vi "MCListbox Controls.vi"(8 "error in":errorcluster, 9 "Item Names":string[][](array[string])=[["localhost", "DMM", "Closed"], ["localhost", "DC Power", "Closed"], ["localhost", "Digitizer", "Closed"]], 11 "MCListBox Ref":refnum<vi>) -> (0 "error out":errorcluster, 3 "dup MCListBox Ref":refnum<vi>)   [LabVIEW 2025, in "Config Tool.lvlib"]
uses:
  Config Tool.lvlib
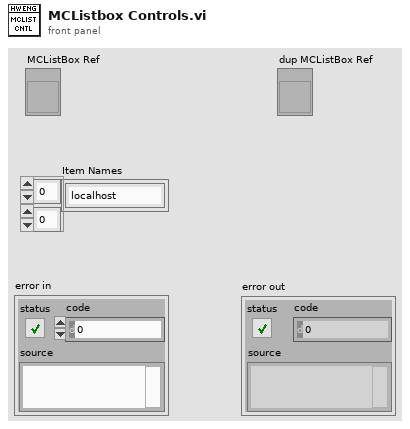
[diagram p1: front panel]
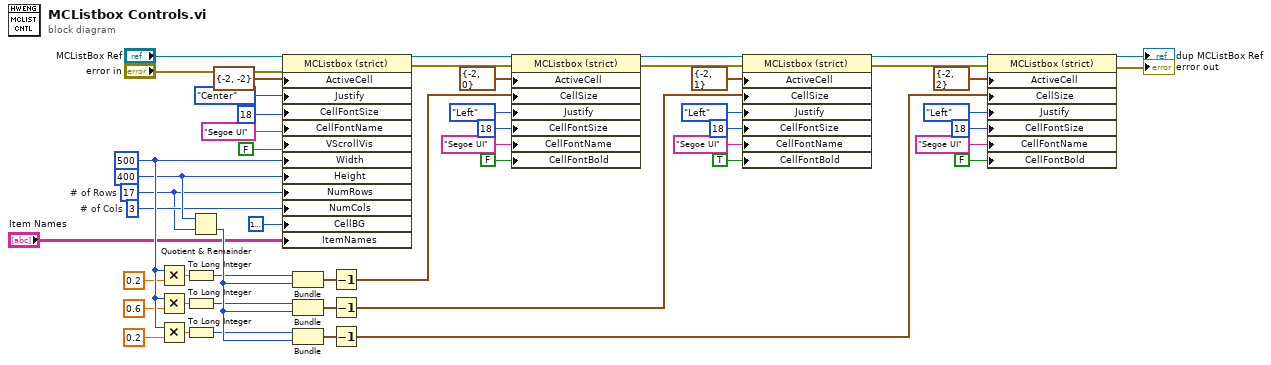
[diagram p0: block diagram]
diagram:
  w35 = u32 400
  w51 = u32 500
  w11 = 3  # # of Cols
  w10 = 17  # # of Rows
  n1 = Multiply(x=w51, y=0.2) -> (x*y=w27:dbl)
  n2 = Multiply(x=w51, y=0.6) -> (x*y=w31:dbl)
  n3 = Multiply(x=w51, y=0.2) -> (x*y=w45:dbl)
  n4 = To Long Integer(number=w27) -> (32bit integer=w28:i32)
  n5 = To Long Integer(number=w31) -> (32bit integer=w30:i32)
  n6 = To Long Integer(number=w45) -> (32bit integer=w46:i32)
  n7 = Quotient & Remainder(x=w35, y=w10) -> (floor(x/y)=w47:u32)  [unwired: 1 out]
  n8 = property on="Property Node" class="MCListbox (strict)"(reference="MCListBox Ref", error in="error in", "ActiveCell"=cluster{"Row":i32, "Column":i32} {"Row"=-2, "Column"=-2} ("Active Cell:Active Cell"), "Justify"=enum16{"Left", "Center", "Right"}."Center" ("Active Cell:Cell Justification"), "CellFontSize"=u32 18 ("Active Cell:Cell Font:Size"), "CellFontName"="Segoe UI" ("Active Cell:Cell Font:Name"), "VScrollVis"=FALSE ("Visible Items:Vertical Scrollbar Visible"), "Width"=w51, "Height"=w35, "NumRows"=w10, "NumCols"=w11, "CellBG"=u32 16777238, "ItemNames"="Item Names") -> (reference out=w13:refnum<vi>, error out=w14:errorcluster)
  n9 = Bundle(w28, w47) -> (w6:cluster{i32, u32})  [unwired: 1 in]
  n10 = Bundle(w30, w47) -> (w32:cluster{i32, u32})  [unwired: 1 in]
  n11 = Bundle(w46, w47) -> (w44:cluster{i32, u32})  [unwired: 1 in]
  n12 = Decrement(x=w6) -> (x-1=w29:cluster{i32, u32})
  n13 = Decrement(x=w32) -> (x-1=w33:cluster{i32, u32})
  n14 = Decrement(x=w44) -> (x-1=w48:cluster{i32, u32})
  n15 = property on="Property Node" class="MCListbox (strict)"(reference=w13, error in=w14, "ActiveCell"=cluster{"Row":i32, "Column":i32} {"Row"=-2, "Column"=0} ("Active Cell:Active Cell"), "CellSize"=w29, "Justify"=enum16{"Left", "Center", "Right"}."Left" ("Active Cell:Cell Justification"), "CellFontSize"=u32 18 ("Active Cell:Cell Font:Size"), "CellFontName"="Segoe UI" ("Active Cell:Cell Font:Name"), "CellFontBold"=FALSE ("Active Cell:Cell Font:Bold")) -> (reference out=w15:refnum<vi>, error out=w16:errorcluster)
  n16 = property on="Property Node" class="MCListbox (strict)"(reference=w15, error in=w16, "ActiveCell"=cluster{"Row":i32, "Column":i32} {"Row"=-2, "Column"=1} ("Active Cell:Active Cell"), "CellSize"=w33, "Justify"=enum16{"Left", "Center", "Right"}."Left" ("Active Cell:Cell Justification"), "CellFontSize"=u32 18 ("Active Cell:Cell Font:Size"), "CellFontName"="Segoe UI" ("Active Cell:Cell Font:Name"), "CellFontBold"=TRUE ("Active Cell:Cell Font:Bold")) -> (reference out=w42:refnum<vi>, error out=w43:errorcluster)
  n17 = property on="Property Node" class="MCListbox (strict)"(reference=w42, error in=w43, "ActiveCell"=cluster{"Row":i32, "Column":i32} {"Row"=-2, "Column"=2} ("Active Cell:Active Cell"), "CellSize"=w48, "Justify"=enum16{"Left", "Center", "Right"}."Left" ("Active Cell:Cell Justification"), "CellFontSize"=u32 18 ("Active Cell:Cell Font:Size"), "CellFontName"="Segoe UI" ("Active Cell:Cell Font:Name"), "CellFontBold"=FALSE ("Active Cell:Cell Font:Bold")) -> (reference out=→"dup MCListBox Ref":refnum<vi>, error out=→"error out":errorcluster)
